vi "combinaison.vi"() -> ()   [LabVIEW 2018]
panel:
  out "Numeric":dbl
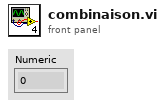
[diagram p1: front panel]
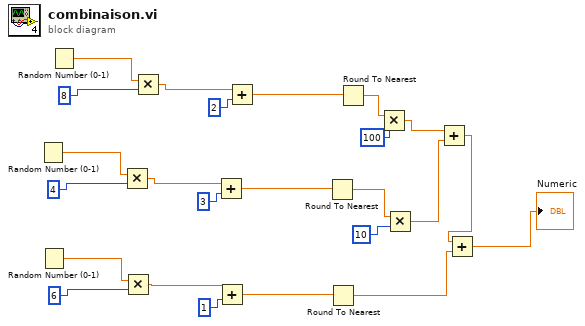
[diagram p0: block diagram]
diagram:
  n1 = Random Number (0-1)() -> (number: 0 to 1=w19:dbl)
  n2 = Random Number (0-1)() -> (number: 0 to 1=w14:dbl)
  n3 = Random Number (0-1)() -> (number: 0 to 1=w24:dbl)
  n4 = Multiply(x=w19, y=4) -> (x*y=w18:dbl)
  n5 = Multiply(x=w14, y=6) -> (x*y=w13:dbl)
  n6 = Multiply(x=w24, y=8) -> (x*y=w23:dbl)
  n7 = Add(x=w18, y=3) -> (x+y=w17:dbl)
  n8 = Add(x=w13, y=1) -> (x+y=w12:dbl)
  n9 = Add(x=w23, y=2) -> (x+y=w22:dbl)
  n10 = Round To Nearest(number=w17) -> (nearest integer value=w6:dbl)
  n11 = Round To Nearest(number=w12) -> (nearest integer value=w8:dbl)
  n12 = Round To Nearest(number=w22) -> (nearest integer value=w7:dbl)
  n13 = Multiply(x=w7, y=100) -> (x*y=w5:dbl)
  n14 = Multiply(x=w6, y=10) -> (x*y=w4:dbl)
  n15 = Add(x=w5, y=w4) -> (x+y=w9:dbl)
  n16 = Add(x=w9, y=w8) -> (x+y=→"Numeric":dbl)
